vi "C4Ftr_release.vi"(0 "c4Ftrs in":refnum<k24>, 11 "error in":errorcluster) -> (15 "error out":errorcluster)   [LabVIEW 2015, in "libC4HdlLV.lvlib"]
uses:
  libC4HdlLV.lvlib
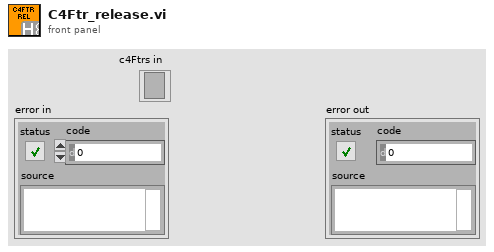
[diagram p1: front panel]
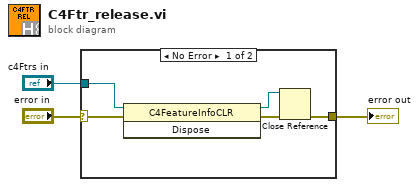
[diagram p0: block diagram]
diagram:
  n1 = case shown="No Error" "error in" {
    selector: "error in" -> [w7 w9]
    tunnel: [w4 w9] -> w2
    tunnel: "c4Ftrs in" -> [w8 _]
    frame No Error {
      n2 = invoke class="C4FeatureInfoCLR" method="Dispose"(reference=w8, error in=w7) -> (reference out=w5:refnum<k24>, error out=w6:errorcluster)  [unwired: 1 in, 1 out]
      n3 = Close Reference(reference=w5, error in (no error)=w6) -> (error out=w4:errorcluster)
    }
    frame Error {
    }
  }
  "error out" <- w2
